vi "Demo.vi"() -> ()   [LabVIEW 2021, in "Autocomplete Textbox.lvlib"]
uses:
  Autocomplete Textbox.lvlib
  Classes/Handle/Init inputs.ctl
  Classes/Handle/Listbox placement.ctl
  SubVIs/Color String Options.ctl
  Classes/Handle/New.vi
  Main Loop.vi
  Classes/Handle/Shutdown.vi
  Classes/Handle/New List.vi
  Classes/Handle/Mouse Down Signal.vi
  Classes/Handle/Handle.lvclass
panel:
  in  "mouse down signal":bool
  in  "String":string
  in  "List":string[](array[string])=["across", "action", "after", "almost", "among", "anathema", "anode", "anopheles", "anorthic", "another", "anothers", "basis", "brother", "cannot", "carrion", "cases", "cerebration", "choice", "circulation", "circulations", "cornering", "cornerstone", "cornerstones", "coronation", "corporation", "corporations", "corridor", "corrosion", "corrosions", "corrupting", "corruption", "dicing", "dicta", "dictaphone", "dictaphones", "dictate", "dictated", "dictates", "dictating", "dictation", "dictations", "dictator", "dictatorial", "dictatorially", "dictators", "dictatorship", "diction", "diction nary", "dictionaries", "dictionary", "dictions", "doctrinaire", "doctrinaires", "doctrinal", "doctrinally", "doctrine", "drift", "drifty", "drippy", "drive", "drivel", "driveled", "drivels", "driven", "driver", "drivers", "drives", "driving", "ducting", "earth", "either", "gar din", "garaging", "garbing", "garbling", "garcon", "garde", "garden", "gardened", "gardener", "gardenia", "gardens", "gardner", "gargling", "goring", "habeas", "habited", "habits", "hebetate", "helicon", "helicopter", "helicopters", "heliotrope", "heliotropes", "heliotropism", "heliport", "hellcat", "hellcats", "hello", "helot", "helotries", "helotry", "helots", "hobbies", "hobbit", "hobbits", "hobblers", "hobbles", "hobbs", "hoboes", "hobos", "holdover", "hothead", "hotline", "hotlines", "hotpoint", "jasmine", "jasmines", "jason", "jaspers", "jests", "km art", "lateen", "lateens", "later", "lateral", "laterals", "lathe", "lather", "lathered", "latherer", "lathers", "lathery", "latter", "latterday", "latterly", "lattices", "leg ht", "legate", "legated", "legatee", "legates", "legato", "legator", "legatos", "leggett", "leghorn", "legit", "letter", "letters", "letterset", "lettersets", "liege", "lieges", "light", "likely", "lines", "lionize", "looking", "lottos", "machete", "machetes", "machine", "machined", "machines", "machinist", "machinists", "mahjong", "mahjongg", "mahoganies", "mahogany", "mahout", "mahouts", "majolica", "major", "majordomo", "majordomos", "majored", "majorette", "majorettes", "majoring", "majorities", "majority", "majors", "manta", "march", "massif", "mastic", "matador", "matadors", "matrimonial", "matrimonially", "matter", "matters", "matzo", "meant", "meccano", "mechanic", "mechanical", "mechanics", "mechanism", "mechanisms", "mechanist", "mechanistic", "mechanistically", "mechanists", "mechanize", "mechanized", "mechanizes", "meteor", "meter", "micas", "micatin", "michael", "michel", "michele", "michelin", "michelle", "michigan", "mickey", "microbic", "micron", "micronuclei", "microsoft", "might", "mighty", "mikes", "million", "mints", "minty", "mocha", "mochas", "mohair", "mohican", "mojave", "monday", "money", "monitor", "monster", "montage", "montana", "monte", "month", "monthly", "months", "monty", "mosaic", "mosaics", "moses", "mossback", "mossier", "mossiest", "mossing", "mosslike", "mossy", "mosts", "mother", "muses", "music", "musical", "musicale", "musicales", "musically", "musicals", "musician", "musicians", "mussily", "mussing", "mussy", "musts", "na iv", "na too", "naiad", "naifs", "nails", "naive", "naively", "naiveness", "naives", "naivete", "naivetes", "naivety", "natatorium", "nation", "national", "nationalism", "nationalist", "nationalistic", "nationalists", "nationalities", "nationality", "nationalize", "nationalizing", "nationally", "nationals", "nations", "neither", "nether", "nether land", "netherlander", "netherlanders", "netherlands", "netherworld", "netherworlds", "netter", "newark", "newborn", "newborns", "newer", "newly", "newmarket", "newport", "newsier", "newsy", "newton", "nicene", "niche", "niched", "niches", "niching", "nicknack", "nicknacks", "night", "nikes", "nikon", "nikons", "nohow", "notepad", "notes", "nothing", "notional", "noway", "palpitation", "palpitations", "parts", "person", "persons", "police", "policed", "polices", "policies", "policy", "poling", "polio", "polish", "polite", "politer", "politest", "politic", "politician", "politicians", "politicizing", "politick", "politicking", "politico", "politicos", "politics", "polities", "polity", "quickly", "reason", "reasons", "right", "rights", "sanative", "schedule", "scheduled", "scheduler", "schedulers", "schedules", "scheduling", "schema", "scheme", "scherzi", "scherzo", "schlep", "schlock", "schneider", "schnook", "schnooks", "scholar", "scholars", "scholl", "school", "schooled", "schooler", "schools", "schooner", "section", "semester", "semite", "senate", "senates", "senator", "senna", "sensate", "sentence", "sentenced", "sentences", "sentries", "she'd", "short", "sight", "situation", "sonant", "stuff", "swaged", "swayed", "swede", "swede en", "sweden", "swedes", "sweeper", "sweet", "sweeten", "sweetened", "sweetener", "sweeteners", "sweetening", "sweetens", "sweeter", "sweetie", "system", "systematic", "systematical", "systematics", "systematize", "systemic", "systemics", "systemize", "systemized", "systemizes", "systemizing", "systemless", "systems", "taurine", "taurines", "tautest", "technical", "touchiest", "toughest", "toughies", "touraine", "toured", "tourism", "tourist", "touristic", "touristically", "tourists", "tourneys", "until", "wander", "wanders", "wiggle", "wiggly", "wight", "wights", "winder", "winders", "windier", "winterkill", "wonder", "wonder full", "wondered", "wonderer", "wonderful", "wonderfully", "wonderfulness", "wonders", "wondrously"]
  in  "Listbox":i32(listbox)
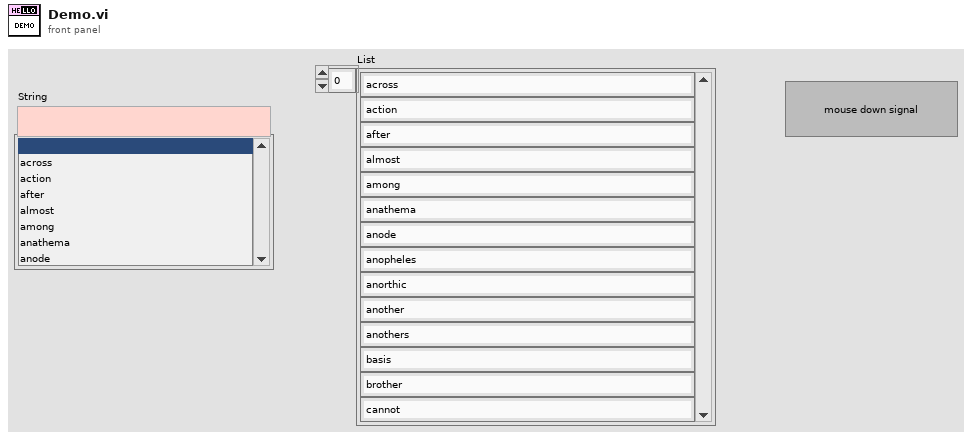
[diagram p1: front panel]
types:
  T1 = typedef "Autocomplete Textbox.lvlib/Handle.lvclass/Listbox placement.ctl" = enum16{"None", "Under String", "Fit to Pane"}
  T2 = typedef "Autocomplete Textbox.lvlib/Handle.lvclass/Init inputs.ctl" = cluster{"List":string[], "max rows":i32, "Listbox placement":T1, "String Color Options":T3}
  T3 = typedef "Autocomplete Textbox.lvlib/Color String Options.ctl" = cluster{"Use? (F)":bool, "Color - Valid":u32, "Color - Invalid":u32, "Allow blank?":bool}
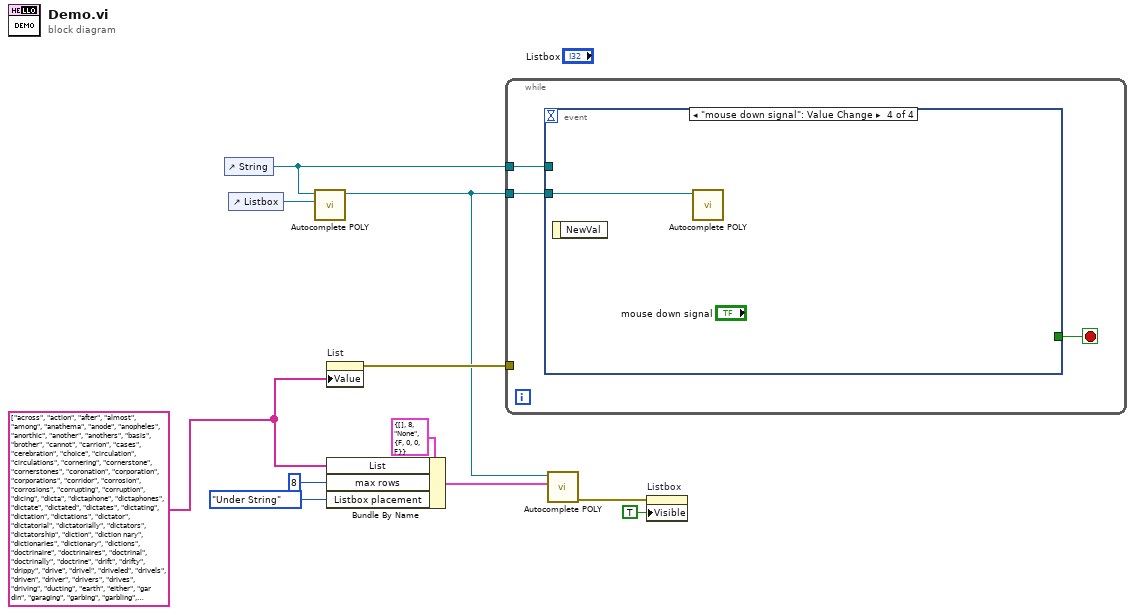
[diagram p0: block diagram]
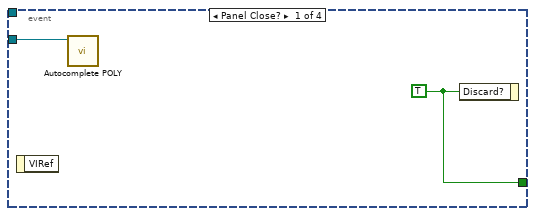
[diagram p2: hidden frame]
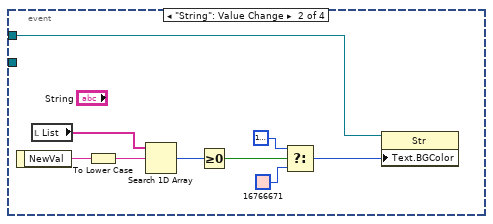
[diagram p3: hidden frame]
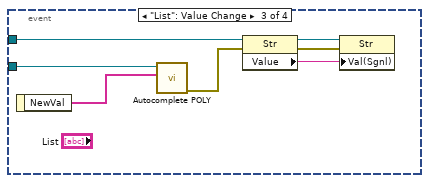
[diagram p4: hidden frame]
diagram:
  w1 = string[] ["across", "action", "after", "almost", "among", "anathema", "anode", "anopheles", "anorthic", "another", "anothers", "basis", "brother", "cannot", "carrion", "cases", "cerebration", "choice", "circulation", "circulations", "cornering", "cornerstone", "cornerstones", "coronation", "corporation", "corporations", "corridor", "corrosion", "corrosions", "corrupting", "corruption", "dicing", "dicta", "dictaphone", "dictaphones", "dictate", "dictated", "dictates", "dictating", "dictation", "dictations", "dictator", "dictatorial", "dictatorially", "dictators", "dictatorship", "diction", "diction nary", "dictionaries", "dictionary", "dictions", "doctrinaire", "doctrinaires", "doctrinal", "doctrinally", "doctrine", "drift", "drifty", "drippy", "drive", "drivel", "driveled", "drivels", "driven", "driver", "drivers", "drives", "driving", "ducting", "earth", "either", "gar din", "garaging", "garbing", "garbling", "garcon", "garde", "garden", "gardened", "gardener", "gardenia", "gardens", "gardner", "gargling", "goring", "habeas", "habited", "habits", "hebetate", "helicon", "helicopter", "helicopters", "heliotrope", "heliotropes", "heliotropism", "heliport", "hellcat", "hellcats", "hello", "helot", "helotries", "helotry", "helots", "hobbies", "hobbit", "hobbits", "hobblers", "hobbles", "hobbs", "hoboes", "hobos", "holdover", "hothead", "hotline", "hotlines", "hotpoint", "jasmine", "jasmines", "jason", "jaspers", "jests", "km art", "lateen", "lateens", "later", "lateral", "laterals", "lathe", "lather", "lathered", "latherer", "lathers", "lathery", "latter", "latterday", "latterly", "lattices", "leg ht", "legate", "legated", "legatee", "legates", "legato", "legator", "legatos", "leggett", "leghorn", "legit", "letter", "letters", "letterset", "lettersets", "liege", "lieges", "light", "likely", "lines", "lionize", "looking", "lottos", "machete", "machetes", "machine", "machined", "machines", "machinist", "machinists", "mahjong", "mahjongg", "mahoganies", "mahogany", "mahout", "mahouts", "majolica", "major", "majordomo", "majordomos", "majored", "majorette", "majorettes", "majoring", "majorities", "majority", "majors", "manta", "march", "massif", "mastic", "matador", "matadors", "matrimonial", "matrimonially", "matter", "matters", "matzo", "meant", "meccano", "mechanic", "mechanical", "mechanics", "mechanism", "mechanisms", "mechanist", "mechanistic", "mechanistically", "mechanists", "mechanize", "mechanized", "mechanizes", "meteor", "meter", "micas", "micatin", "michael", "michel", "michele", "michelin", "michelle", "michigan", "mickey", "microbic", "micron", "micronuclei", "microsoft", "might", "mighty", "mikes", "million", "mints", "minty", "mocha", "mochas", "mohair", "mohican", "mojave", "monday", "money", "monitor", "monster", "montage", "montana", "monte", "month", "monthly", "months", "monty", "mosaic", "mosaics", "moses", "mossback", "mossier", "mossiest", "mossing", "mosslike", "mossy", "mosts", "mother", "muses", "music", "musical", "musicale", "musicales", "musically", "musicals", "musician", "musicians", "mussily", "mussing", "mussy", "musts", "na iv", "na too", "naiad", "naifs", "nails", "naive", "naively", "naiveness", "naives", "naivete", "naivetes", "naivety", "natatorium", "nation", "national", "nationalism", "nationalist", "nationalistic", "nationalists", "nationalities", "nationality", "nationalize", "nationalizing", "nationally", "nationals", "nations", "neither", "nether", "nether land", "netherlander", "netherlanders", "netherlands", "netherworld", "netherworlds", "netter", "newark", "newborn", "newborns", "newer", "newly", "newmarket", "newport", "newsier", "newsy", "newton", "nicene", "niche", "niched", "niches", "niching", "nicknack", "nicknacks", "night", "nikes", "nikon", "nikons", "nohow", "notepad", "notes", "nothing", "notional", "noway", "palpitation", "palpitations", "parts", "person", "persons", "police", "policed", "polices", "policies", "policy", "poling", "polio", "polish", "polite", "politer", "politest", "politic", "politician", "politicians", "politicizing", "politick", "politicking", "politico", "politicos", "politics", "polities", "polity", "quickly", "reason", "reasons", "right", "rights", "sanative", "schedule", "scheduled", "scheduler", "schedulers", "schedules", "scheduling", "schema", "scheme", "scherzi", "scherzo", "schlep", "schlock", "schneider", "schnook", "schnooks", "scholar", "scholars", "scholl", "school", "schooled", "schooler", "schools", "schooner", "section", "semester", "semite", "senate", "senates", "senator", "senna", "sensate", "sentence", "sentenced", "sentences", "sentries", "she'd", "short", "sight", "situation", "sonant", "stuff", "swaged", "swayed", "swede", "swede en", "sweden", "swedes", "sweeper", "sweet", "sweeten", "sweetened", "sweetener", "sweeteners", "sweetening", "sweetens", "sweeter", "sweetie", "system", "systematic", "systematical", "systematics", "systematize", "systemic", "systemics", "systemize", "systemized", "systemizes", "systemizing", "systemless", "systems", "taurine", "taurines", "tautest", "technical", "touchiest", "toughest", "toughies", "touraine", "toured", "tourism", "tourist", "touristic", "touristically", "tourists", "tourneys", "until", "wander", "wanders", "wiggle", "wiggly", "wight", "wights", "winder", "winders", "windier", "winterkill", "wonder", "wonder full", "wondered", "wonderer", "wonderful", "wonderfully", "wonderfulness", "wonders", "wondrously"] ("words")
  n1 = control-ref of="String"() -> (w6:refnum<vi>)
  n2 = control-ref of="Listbox"() -> (w5:refnum<vi>)
  n3 = call-poly "Autocomplete POLY.vi"("Listbox"=w5, "String"=w6) -> ("Handle out"=w8:refnum<class "Handle.lvclass">)  [unwired: 8 in, 1 out]
  n4 = property on="List" class="Arr (strict)"("Value"=w1) -> (error out=w9:errorcluster)  [unwired: 2 in, 1 out]
  n5 = Bundle By Name(cluster=T2 {"List"=[], "max rows"=8, "Listbox placement"=enum."None", "String Color Options"={"Use? (F)"=FALSE, "Color - Valid"=0, "Color - Invalid"=0, "Allow blank?"=FALSE}} ("Init options"), "List"=w1, "max rows"=8, "Listbox placement"=Listbox_placement."Under String") -> (w7:T2)
  n6 = while {
    tunnel: w8 -> [w13]
    tunnel: w6 -> [w12]
    tunnel: w9 -> [_]
    stop <- w14 stop-if-true
    n7 = event shown="[3] \"mouse down signal\": Value Change" {
      selector: _ -> [_ _ _ _]
      dyn-events: _ -> [_ _ _ _]
      timeout: _ -> [_ _ _ _]
      tunnel: [w16 _ _ _] -> w14
      tunnel: w13 -> [w15 _ w28 w33]
      tunnel: w12 -> [_ w18 w32 _]
      event Panel Close? {
        w16 = TRUE ("Discard?")
        n8 = event-data() -> ()  [unwired: 1 in, 1 out]
        n9 = call-poly "Autocomplete POLY.vi"("Handle in"=w15) -> ()  [unwired: 9 in, 2 out]
        n10 = event-data("Discard?"=w16) -> ()  [unwired: 1 in, 1 out]
      }
      event "String": Value Change {
        n11 = event-data() -> ("NewVal"=w25:string)  [unwired: 1 in]
        n12 = local read "List"() -> (w17:string[])
        n13 = To Lower Case(string=w25) -> (all lower case string=w24:string)
        n14 = Search 1D Array(1D array=w17, element=w24) -> (index of element=w23:i32)  [unwired: 1 in]
        n15 = Greater Or Equal To 0?(x=w23) -> (x >= 0?=w19:bool)
        n16 = Select(t=u32 16777226, s=w19, f=u32 16766671) -> (s? t:f=w22:u32)
        n17 = property class="Str"(reference=w18, "Text.BGColor"=w22) -> ()  [unwired: 1 in, 2 out]
      }
      event "List": Value Change {
        n18 = event-data() -> ("NewVal"=w27:string[])  [unwired: 1 in]
        n19 = call-poly "Autocomplete POLY.vi"("List"=w27, "Handle in"=w28) -> ("error out"=w26:errorcluster)  [unwired: 8 in, 1 out]
        n20 = property class="Str"(reference=w32, error in=w26) -> (reference out=w31:refnum<vi>, error out=w30:errorcluster, "Value"=w29:string)
        n21 = property class="Str"(reference=w31, error in=w30, "Val(Sgnl)"=w29) -> ()  [unwired: 2 out]
      }
      event "mouse down signal": Value Change {
        n22 = event-data() -> ()  [unwired: 1 in, 1 out]
        n23 = call-poly "Autocomplete POLY.vi"("Handle in"=w33) -> ()  [unwired: 9 in, 2 out]
      }
    }
  }
  n24 = call-poly "Autocomplete POLY.vi"("Init options"=w7, "Handle"=w8) -> ("error out"=w4:errorcluster)  [unwired: 7 in, 2 out]
  n25 = property on="Listbox" class="LstBox (strict)"(error in=w4, "Visible"=TRUE) -> ()  [unwired: 1 in, 2 out]
